vi "RESTful RoutingType To Text.vi"(1 "Routing Type":T1=enum."Static") -> (0 "Boolean Text":string)   [LabVIEW 2020]
uses:
  <vilib>/AppBuilder/AB_Classes/RESTful/AB_RESTful_RoutingType.ctl
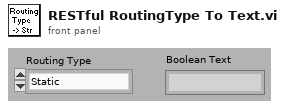
[diagram p1: front panel]
types:
  T1 = typedef "AB_RESTful_RoutingType.ctl" = enum32{"Method", "Static"}
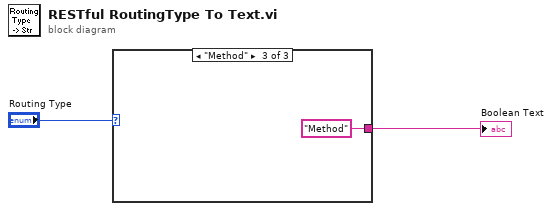
[diagram p0: block diagram]
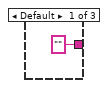
[diagram p2: hidden frame]
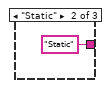
[diagram p3: hidden frame]
diagram:
  n1 = case shown="\"Method\"" "Routing Type" {
    tunnel: ["" ("Boolean Text") "Static" ("Boolean Text") "Method" ("Boolean Text")] -> w2
    frame Default {
    }
    frame "Static" {
    }
    frame "Method" {
    }
  }
  "Boolean Text" <- w2
